vi "Untitled 3 (SubVI).vi"(4 "radians":dbl) -> (1 "Numeric":dbl)   [LabVIEW 2015]
panel:
  in  "Boolean":bool
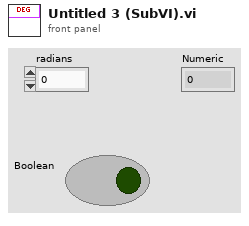
[diagram p1: front panel]
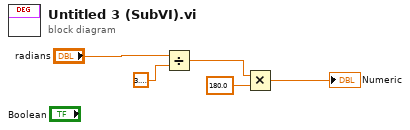
[diagram p0: block diagram]
diagram:
  n1 = Divide(x="radians", y=3.141592653589793) -> (x/y=w2:dbl)
  n2 = Multiply(x=w2, y=180.0) -> (x*y=→"Numeric":dbl)
